vi "Execution Loop Start.vi"(8 "error in (no error)":errorcluster, 10 "Execution in":refnum<data-value>, 11 "Project in":refnum<class "Project.lvclass">) -> (0 "error out":errorcluster, 2 "Execution out":refnum<data-value>, 3 "Project out":refnum<class "Project.lvclass">)   [LabVIEW 2015, in "Project.lvclass"]
uses:
  Project.lvclass
  Execution.lvclass
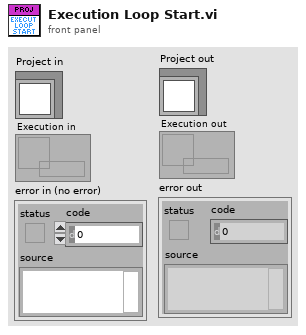
[diagram p1: front panel]
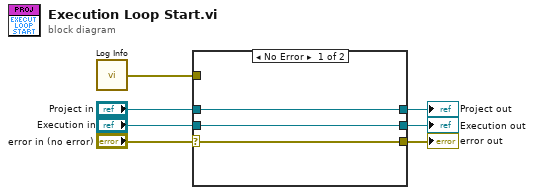
[diagram p0: block diagram]
diagram:
  n1 = call "Log Info.vi"() -> ("error out"=w3:errorcluster)  [unwired: 5 in]
  n2 = case shown="No Error" "error in (no error)" {
    selector: "error in (no error)" -> [w9 w13]
    tunnel: [w9 w13] -> w6
    tunnel: [w10 w12] -> w4
    tunnel: "Project in" -> [w10 w12]
    tunnel: w3 -> [_ _]
    tunnel: "Execution in" -> [w8 w11]
    tunnel: [w8 w11] -> w1
    frame No Error {
    }
    frame Error {
    }
  }
  "error out" <- w6
  "Project out" <- w4
  "Execution out" <- w1
